vi "Error Strings Global.vi"() -> ()   [LabVIEW 2020]
panel:
  out "5057":string="Invalid measurement metadata. The following parameter names in `Get Type Specializations.vi` do not match any controls in  `Measurement Configuration.ctl`:"
  out "5056":string="Timed out waiting for discovery service to start."
  out "5055":string="Failed to read the discovery service key file."
  out "5054":string="Failed to get the discovery service key file size."
  out "5053":string="Failed to read the discovery service key file.\nEnsure that the discovery service is running."
  out "5052":string="This method must be overridden"
  out "5051":string="LabVIEW cluster contains a type '%s' which is not supported in gRPC."
  out "5050":string="The data type of the following controls are not supported by the Measurement Service.\n\n%s"
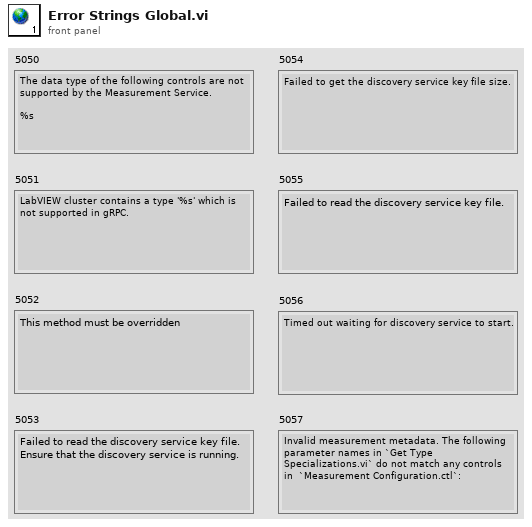
[diagram p1: front panel]
diagram:
